vi "connection.create_connection.vi"(7 "description":string, 8 "error in":errorcluster, 9 "nominalDataSourceRid":string, 10 "name":string, 11 "Nominal Client in":refnum<class "Nominal Client.lvclass">) -> (0 "error out":errorcluster, 1 "Response":string, 2 "response":T1, 3 "Nominal Client out":refnum<class "Nominal Client.lvclass">)   [LabVIEW 2020, in "Nominal Client.lvclass"]
doc: "Creates a new connection.\n\nIf the ID is not unique, a timestamp will be added to the ID."
uses:
  Nominal Client.lvclass
  301638a4-f299-4835-8683-15cfc56d6fd6.vi
  28804fc9-aee6-4b6e-ba11-1ba961eefadd.vi
  <vilib>/JDP Science/JSONtext/Variant to JSON Text.vi
  <vilib>/JDP Science/JSONtext/Get all Object Items.vi
  <vilib>/JDP Science/JSONtext/Set Multiple Object Items.vi
  <vilib>/JDP Science/JSONtext/JSON text to Variant.vi
  <vilib>/JDP Science/JSONtext/LVClass Serializer/JSONtext LVClass Serializer.lvclass
  Nominal Client.lvclass/Nominal Client.ctl
  <vilib>/JDP Science/JSONtext/JSONtext.lvlib
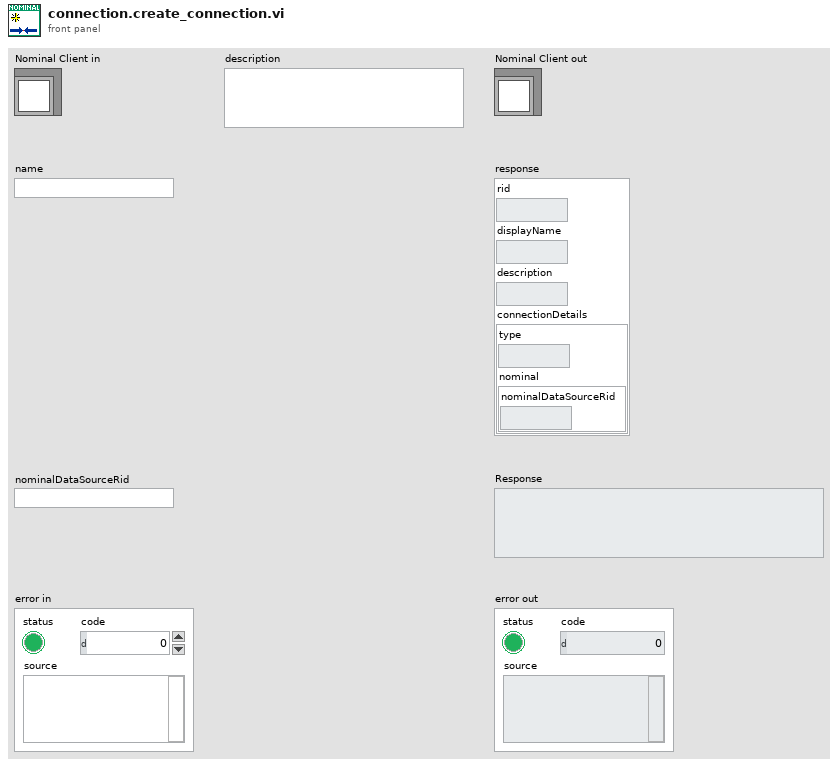
[diagram p1: front panel]
types:
  T1 = cluster{"rid":string, "displayName":string, "description":string, "connectionDetails":cluster{"type":string, "nominal":cluster{"nominalDataSourceRid":string}}}
  T2 = cluster{"type":string, "nominal":cluster{"nominalDataSourceRid":string}}
  T3 = cluster{"name":string, "description":string, "connectionDetails":cluster{"type":string, "nominal":cluster{"nominalDataSourceRid":string}}}
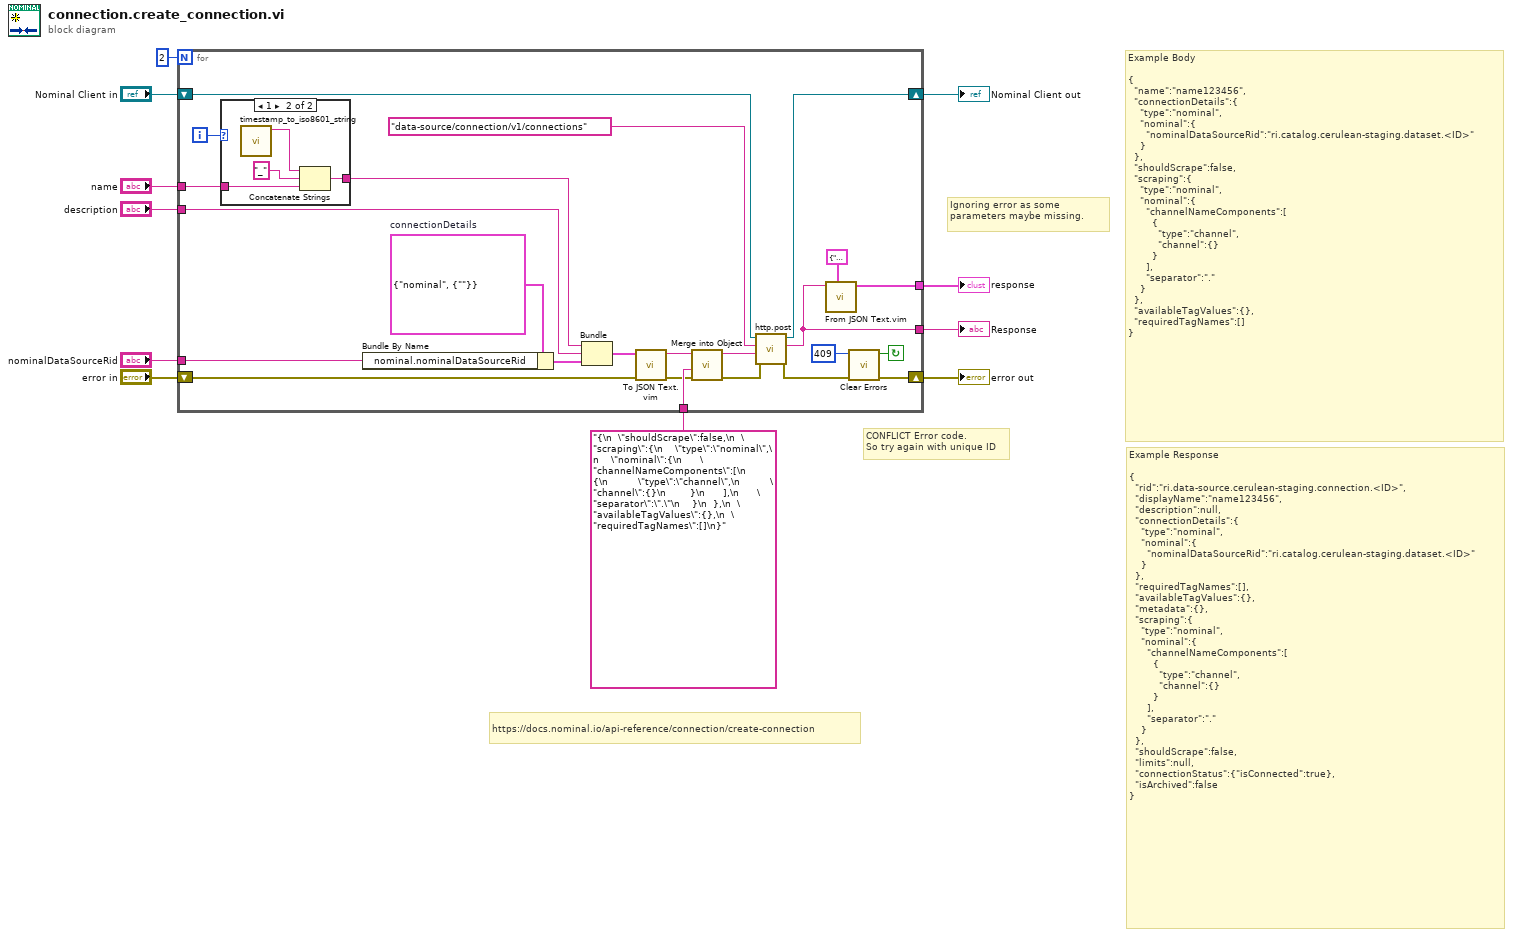
[diagram p0: block diagram]
diagram:
  # "CONFLICT Error code.\nSo try again with unique ID"
  # "https://docs.nominal.io/api-reference/connection/create-connection"
  # "Ignoring error as some parameters maybe missing."
  # "Example Response\n\n{\n  \"rid\":\"ri.data-source.cerulean-staging.connection.<ID>\",\n  \"displayName\":\"name123456\",\n  \"description\":null,\n  \"connectionDetails\":{\n    \"type\":\"nominal\",\n    \"nominal\":{\n      \"nominalDataSourceRid\":\"ri.catalog.cerulean-staging.dataset.<ID>\"\n    }\n  },\n  \"requiredTagNames\":[],\n  \"availableTagValues\":{},\n  \"metadata\":{},\n  \"scraping\":{\n    \"type\":\"nominal\",\n    \"nominal\":{\n      \"channelNameComponents\":[\n        {\n          \"type\":\"channel\",\n          \"channel\":{}\n        }\n      ],\n      \"separator\":\".\"\n    }\n  },\n  \"shouldScrape\":false,\n  \"limits\":null,\n  \"connectionStatus\":{\"isConnected\":true},\n  \"isArchived\":false\n}"
  # "Example Body\n\n{\n  \"name\":\"name123456\",\n  \"connectionDetails\":{\n    \"type\":\"nominal\",\n    \"nominal\":{\n      \"nominalDataSourceRid\":\"ri.catalog.cerulean-staging.dataset.<ID>\"\n    }\n  },\n  \"shouldScrape\":false,\n  \"scraping\":{\n    \"type\":\"nominal\",\n    \"nominal\":{\n      \"channelNameComponents\":[\n        {\n          \"type\":\"channel\",\n          \"channel\":{}\n        }\n      ],\n      \"separator\":\".\"\n    }\n  },\n  \"availableTagValues\":{},\n  \"requiredTagNames\":[]\n}"
  n1 = for {
    N: 2 -> [_]
    tunnel: "nominalDataSourceRid" -> [w32]
    tunnel: [w20] -> w4
    tunnel: "name" -> [w13]
    tunnel: "description" -> [w19]
    shift-right: [w28] -> w7
    shift-left: "Nominal Client in" -> [w35]
    shift-right: [w16] -> w8
    shift-left: "error in" -> [w30]
    tunnel: "{\n  \"shouldScrape\":false,\n  \"scraping\":{\n    \"type\":\"nominal\",\n    \"nominal\":{\n      \"channelNameComponents\":[\n        {\n          \"type\":\"channel\",\n          \"channel\":{}\n        }\n      ],\n      \"separator\":\".\"\n    }\n  },\n  \"availableTagValues\":{},\n  \"requiredTagNames\":[]\n}" ("Request body") -> [w27]
    tunnel: [w22] -> w5
    i -> [w14]
    stop <- w18 continue-if-true
    w34 = T2 {"type"="nominal", "nominal"={"nominalDataSourceRid"=""}}  # connectionDetails
    n2 = case shown="1" w14 {
      tunnel: w13 -> [w36 w40]
      tunnel: [w36 w39] -> w12
      frame 0, Default {
      }
      frame 1 {
        n3 = call "timestamp_to_iso8601_string.vi"() -> ("ISO8601 UTC DateTime"=w37:string)  [unwired: 11 in]
        n4 = Concatenate Strings(w37, "_" ("string"), w40) -> (w39:string)
      }
    }
    n5 = Bundle By Name(cluster=w34, "nominal.nominalDataSourceRid"=w32) -> (w33:T2)
    n6 = Bundle("name"=w12, "description"=w19, "connectionDetails"=w33) -> (w31:T3)  [unwired: 1 in]
    n7 = call "To JSON Text.vim"("error in (no error)"=w30, "Anything"=w31) -> ("error out"=w24:errorcluster, "<JSON>"=w26:string)  [unwired: 8 in]
    n8 = call <vilib>:"Merge into Object.vi"("error in (no error)"=w24, "JSON Object to Merge"=w27, "JSON"=w26) -> ("error out"=w23:errorcluster, "<JSON>"=w25:string)  [unwired: 6 in]
    n9 = call "http.post.vi"("error in"=w23, "Request body"=w25, "Path"="data-source/connection/v1/connections", "Nominal Client in"=w35) -> ("error out"=w17:errorcluster, "Response"=w22:string, "Nominal Client out"=w28:refnum<class "Nominal Client.lvclass">)  [unwired: 4 in, 1 out]
    n10 = call "From JSON Text.vim"("Data Type and Default Value"=T1 {"rid"="", "displayName"="", "description"="", "connectionDetails"={"type"="", "nominal"={"nominalDataSourceRid"=""}}} ("response"), "JSON"=w22) -> ("Data out"=w20:T1)  [unwired: 8 in, 1 out]
    n11 = call <vilib>:"Clear Errors.vi"("error in (no error)"=w17, "specific error code to clear (0: all)"=409) -> ("error out"=w16:errorcluster, "specific error cleared?"=w18:bool)  [unwired: 4 in]
  }
  "Nominal Client out" <- w7
  "error out" <- w8
  "Response" <- w5
  "response" <- w4
